vi "ARCH_EDITOR_prepare_UPDATE_transaction.vi"(7 "nmb_of_top_rows (all)":i32, 8 "error_in":errorcluster, 10 "selected_record":i32, 11 "ARCH_EDIT_records":string[][](array[string])) -> (0 "error_out":errorcluster, 3 "UPDATE_transaction":string[](array[string]))   [LabVIEW 2019]
uses:
  FGV/login/FGV_login.ctl
  FGV/ARCH_EDITOR_records_display/FGV_ARCH_EDITOR_records_display.ctl
  <userlib>/_OpenG.lib/array/array.llb/Filter 1D Array (String)__ogtk.vi
  <userlib>/_OpenG.lib/array/array.llb/Delete Elements from 1D Array (String)__ogtk.vi
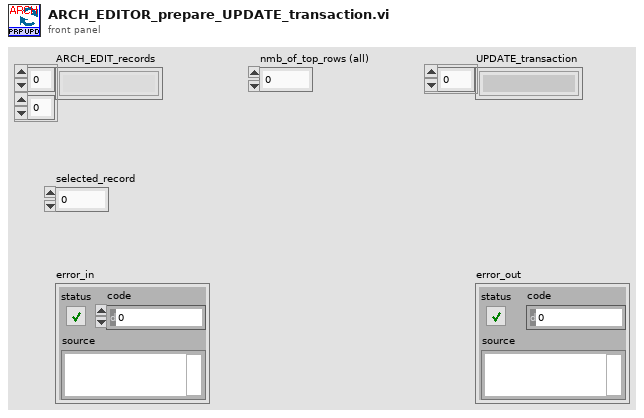
[diagram p1: front panel]
types:
  T1 = typedef "FGV_ARCH_EDITOR_records_display.ctl" = enum16{"initialize", "set_arch_cfg_tables_names", "set_station_number", "set_type_filter", "set_headers", "set_records", "get_arch_cfg_table_name", "get_arch_cfg_hist_table_name", "get_station_number", "get_type_filter", "get_headers", "get_uneditable_columns", "get_all_info", "record_added?", "record_inserted?", "record_edited?", "record_updated?", "record_deleted?", "discard_changes"}
  T2 = typedef "FGV_login.ctl" = enum16{"initialize", "login", "logout", "get_login_info"}
  T3 = typedef "ARCH_EDITOR_all_info.ctl" = cluster{"station_number":string, "type_filter":string, "archivisation_cfg_table":string, "archivisation_cfg_history":string, "column_names":string[], "uneditable_columns":string[], "uneditable_columns":i32[], "editable_columns":i32[], "values_in_database":string[][], "size":cluster{"columns":i32, "SQL_rows":i32, "disp_rows":i32}, "ARCH_record_states":T4[]}
  T4 = typedef "SQL_record_states.ctl" = enum16{"Equal", "Added", "Edited", "Deleted"}
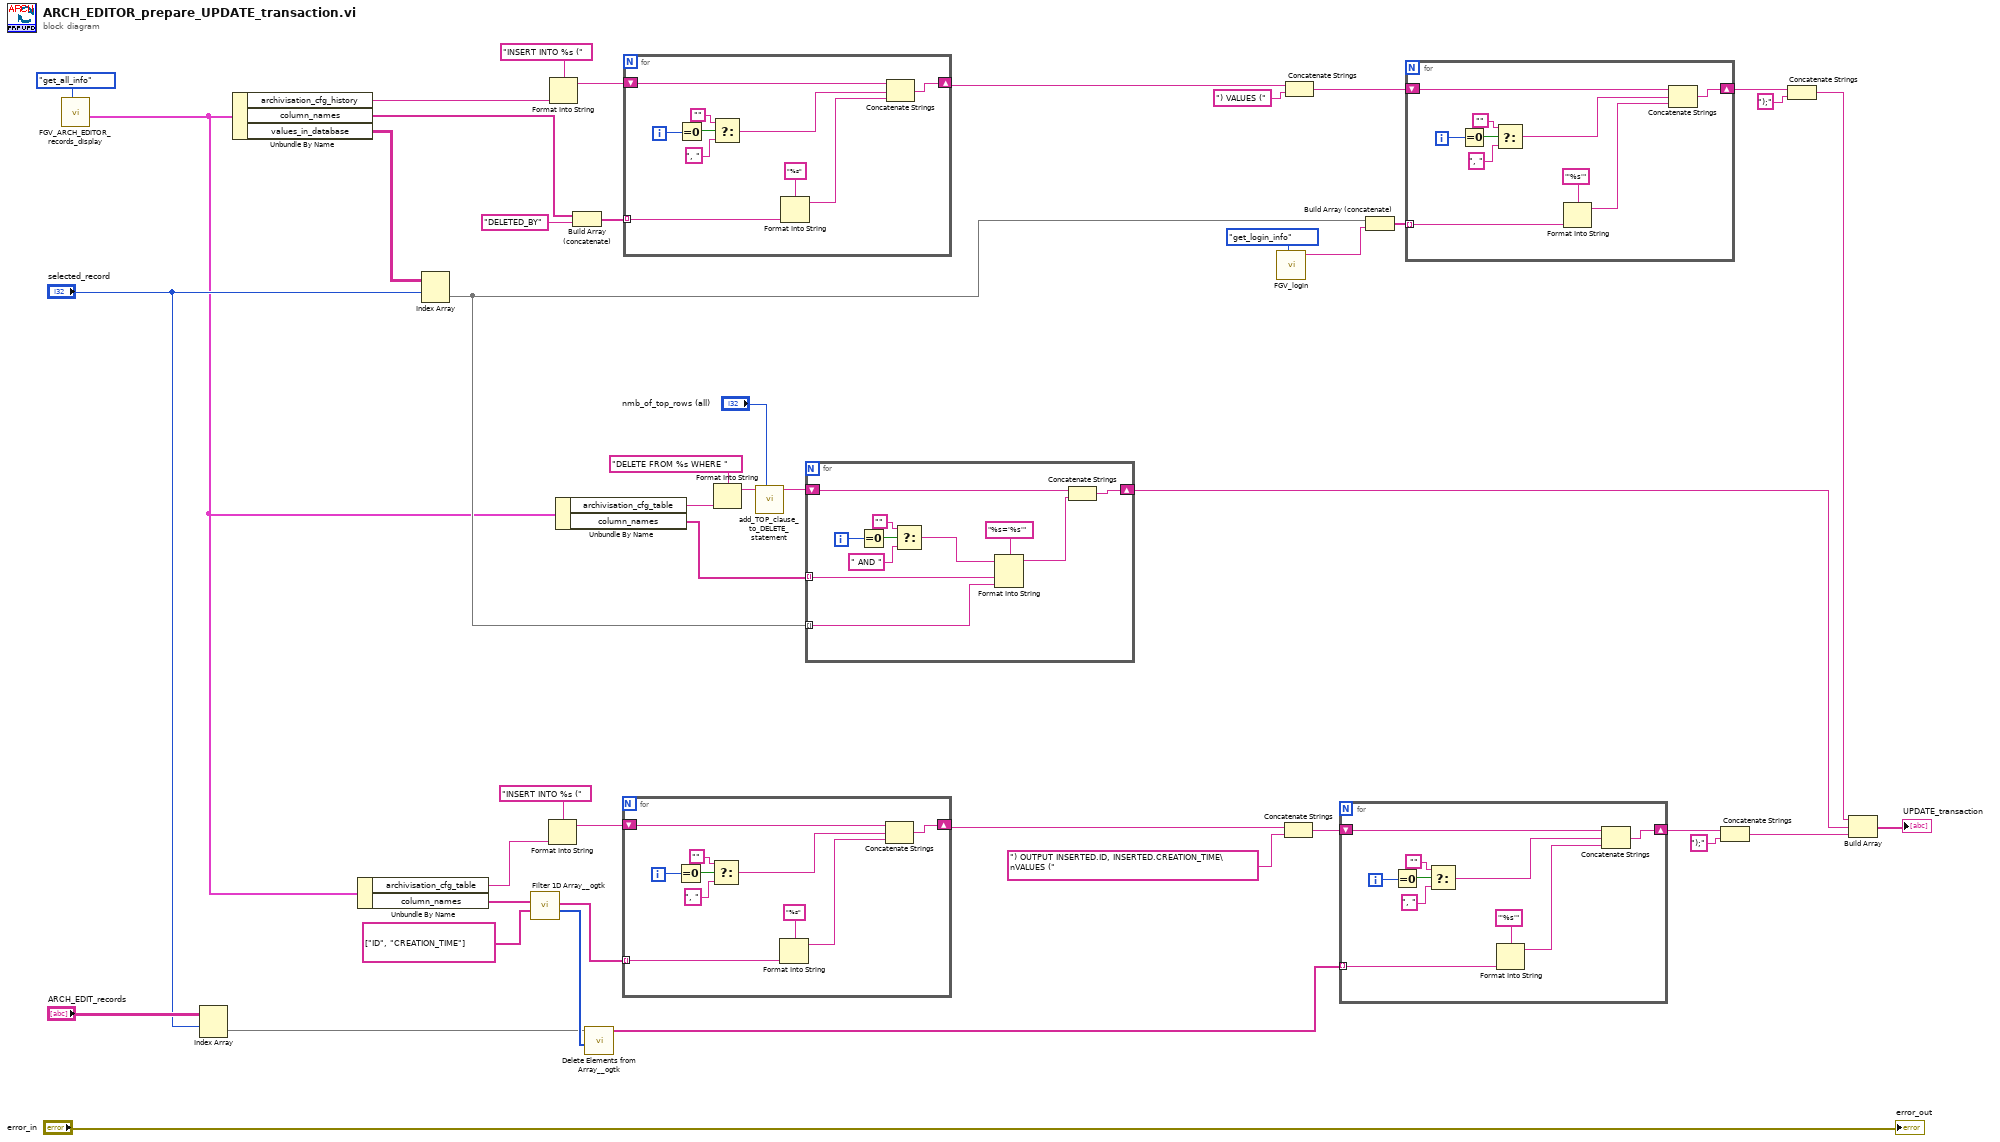
[diagram p0: block diagram]
diagram:
  n1 = call "FGV_ARCH_EDITOR_records_display.vi"("options"=FGV_ARCH_EDITOR_records_display."get_all_info") -> ("all_info"=w3:T3)  [unwired: 7 in, 3 out]
  n2 = Index Array(array="ARCH_EDIT_records", index (row)="selected_record") -> (element=w2:string[])  [unwired: 1 in]
  n3 = Unbundle By Name(w3) -> ("archivisation_cfg_history"=w36:string, "column_names"=w35:string[], "values_in_database"=w29:string[][])
  n4 = Unbundle By Name(w3) -> ("archivisation_cfg_table"=w5:string, "column_names"=w6:string[])
  n5 = Index Array(array=w29, index (row)="selected_record") -> (element=w19:string[])  [unwired: 1 in]
  n6 = call-poly <userlib>:"Filter 1D Array__ogtk.vi"("items to filter"=string[] ["ID", "CREATION_TIME"], "array"=w6) -> ("filtered item indices"=w10:i32[], "filtered array"=w12:string[])  [unwired: 4 in]
  n7 = Format Into String(format string="INSERT INTO %s (", w5) -> (resulting string=w15:string)  [unwired: 2 in, 1 out]
  n8 = Format Into String(format string="INSERT INTO %s (", w36) -> (resulting string=w41:string)  [unwired: 2 in, 1 out]
  n9 = Unbundle By Name(w3) -> ("archivisation_cfg_table"=w21:string, "column_names"=w22:string[])
  n10 = Build Array (concatenate)(w35, "DELETED_BY" ("reference_history")) -> (w34:string[])
  n11 = call-poly <userlib>:"Delete Elements from Array__ogtk.vi"("indices"=w10, "array"=w2) -> ("array w/ subset deleted"=w9:string[])  [unwired: 8 in, 1 out]
  n12 = for {
    tunnel: w12 -> [w48] mode=indexing
    shift-right: [w50] -> w16
    shift-left: w15 -> [w51]
    i -> [w55]
    n13 = Equal To 0?(x=w55) -> (x = 0?=w54:bool)
    n14 = Select(t="", s=w54, f=", ") -> (s? t:f=w49:string)
    n15 = Format Into String(format string="%s", w48) -> (resulting string=w47:string)  [unwired: 2 in, 1 out]
    n16 = Concatenate Strings(w51, w49, w47) -> (w50:string)
  }
  n17 = for {
    tunnel: w34 -> [w58] mode=indexing
    shift-right: [w60] -> w43
    shift-left: w41 -> [w61]
    i -> [w65]
    n18 = Equal To 0?(x=w65) -> (x = 0?=w64:bool)
    n19 = Select(t="", s=w64, f=", ") -> (s? t:f=w59:string)
    n20 = Format Into String(format string="%s", w58) -> (resulting string=w57:string)  [unwired: 2 in, 1 out]
    n21 = Concatenate Strings(w61, w59, w57) -> (w60:string)
  }
  n22 = Format Into String(format string="DELETE FROM %s WHERE ", w21) -> (resulting string=w24:string)  [unwired: 2 in, 1 out]
  n23 = call "add_TOP_clause_to_DELETE_statement.vi"("nmb_of_top_rows (all)"="nmb_of_top_rows (all)", "DELETE_statement_in"=w24) -> ("DELETE_statement_out"=w25:string)  [unwired: 8 in, 1 out]
  n24 = for {
    tunnel: w19 -> [w68] mode=indexing
    tunnel: w22 -> [w69] mode=indexing
    shift-right: [w66] -> w17
    shift-left: w25 -> [w72]
    i -> [w76]
    n25 = Equal To 0?(x=w76) -> (x = 0?=w75:bool)
    n26 = Select(t="", s=w75, f=" AND ") -> (s? t:f=w70:string)
    n27 = Format Into String(format string="%s='%s'", initial string=w70, w69, w68) -> (resulting string=w67:string)  [unwired: 1 in, 1 out]
    n28 = Concatenate Strings(w72, w67) -> (w66:string)
  }
  n29 = call "FGV_login.vi"("options"=FGV_login."get_login_info") -> ("username_out"=w30:string)  [unwired: 8 in, 2 out]
  n30 = Concatenate Strings(w16, ") OUTPUT INSERTED.ID, INSERTED.CREATION_TIME\nVALUES (" ("string")) -> (w11:string)
  n31 = Concatenate Strings(w43, ") VALUES (" ("string")) -> (w39:string)
  n32 = for {
    tunnel: w9 -> [w79] mode=indexing
    shift-right: [w81] -> w7
    shift-left: w11 -> [w82]
    i -> [w86]
    n33 = Equal To 0?(x=w86) -> (x = 0?=w85:bool)
    n34 = Select(t="", s=w85, f=", ") -> (s? t:f=w80:string)
    n35 = Format Into String(format string="'%s'", w79) -> (resulting string=w78:string)  [unwired: 2 in, 1 out]
    n36 = Concatenate Strings(w82, w80, w78) -> (w81:string)
  }
  n37 = Build Array (concatenate)(w19, w30) -> (w32:string[])
  n38 = for {
    tunnel: w32 -> [w89] mode=indexing
    shift-right: [w91] -> w37
    shift-left: w39 -> [w92]
    i -> [w96]
    n39 = Equal To 0?(x=w96) -> (x = 0?=w95:bool)
    n40 = Select(t="", s=w95, f=", ") -> (s? t:f=w90:string)
    n41 = Format Into String(format string="'%s'", w89) -> (resulting string=w88:string)  [unwired: 2 in, 1 out]
    n42 = Concatenate Strings(w92, w90, w88) -> (w91:string)
  }
  n43 = Concatenate Strings(w7, ");" ("string")) -> (w4:string)
  n44 = Concatenate Strings(w37, ");" ("string")) -> (w18:string)
  n45 = Build Array(w18, w17, w4) -> (→"UPDATE_transaction":string[])
  "error_out" <- "error_in"
